vi "Tx Disable channel logic 1ch 4SPC.vi"(6 "ready for output":bool, 9 "input valid":bool, 10 "data in":u32[](array[numeric])=[0, 0, 0, 0, 0, 0, 0, 0, 0, 0, 0, 0, 0, 0, 0, 0]) -> (0 "enable new data":bool, 1 "output valid":bool, 2 "data out":u32[](array[numeric]))   [LabVIEW 2025, in "niUSRP Stream Control (DMA) v1 FPGA.lvclass"]
uses:
  niUSRP Stream Control (DMA) v1 FPGA.lvclass
  niUSRP Stream Control (DMA) v1 FPGA.lvclass/niUSRP Stream Control (DMA) v1 FPGA.ctl
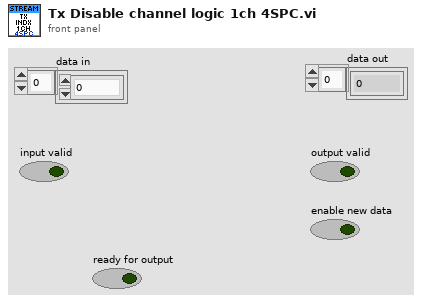
[diagram p1: front panel]
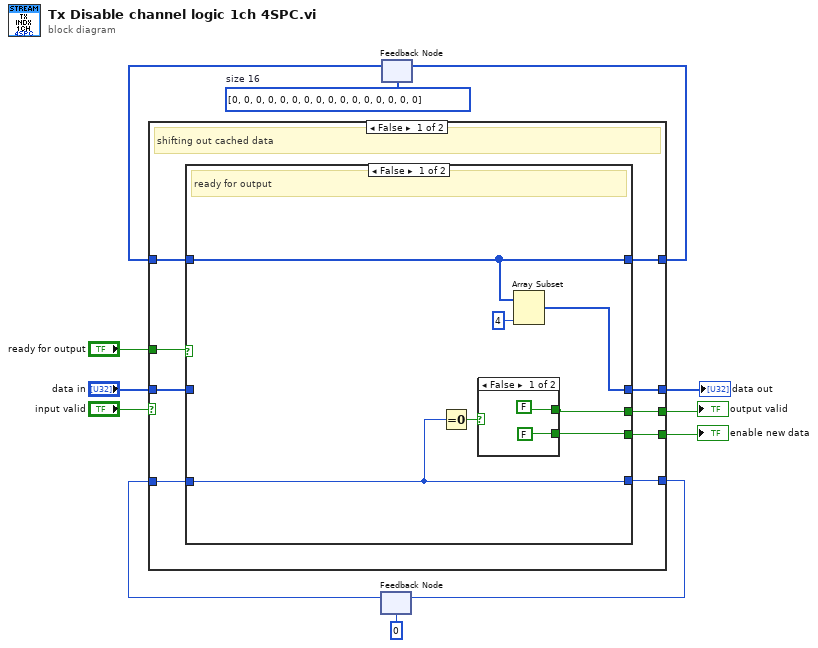
[diagram p0: block diagram]
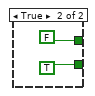
[diagram p2: hidden frame]
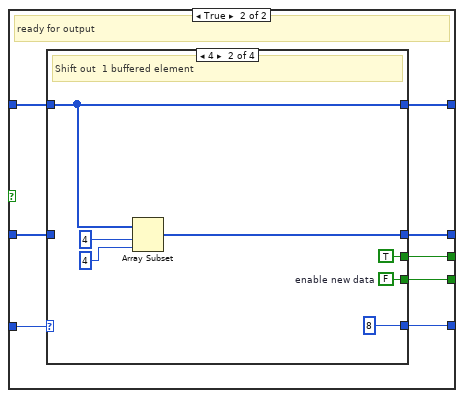
[diagram p3: hidden frame]
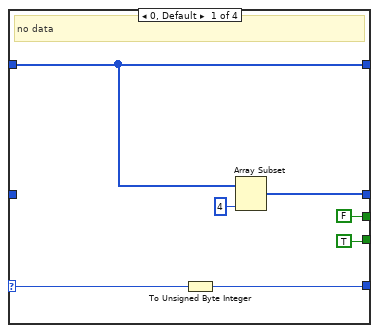
[diagram p4: hidden frame]
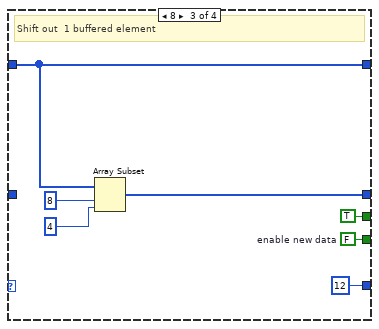
[diagram p5: hidden frame]
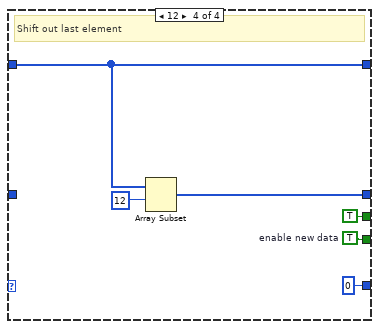
[diagram p6: hidden frame]
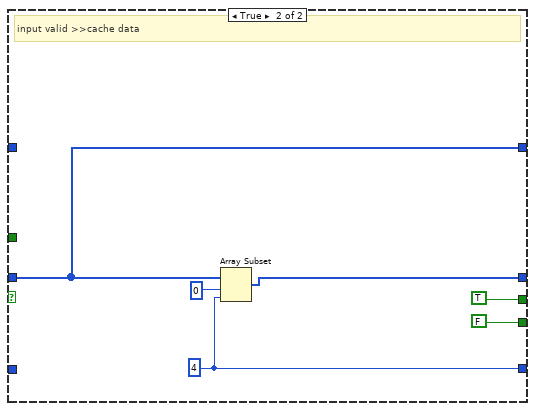
[diagram p7: hidden frame]
diagram:
  w6 = u32[] [0, 0, 0, 0, 0, 0, 0, 0, 0, 0, 0, 0, 0, 0, 0, 0]  # size 16
  n1 = feedback #1(u8 0) -> (w2:u8)
  n2 = feedback #2(w6) -> (w5:u32[])
  n3 = case shown="False" "input valid" {
    tunnel: [w21 TRUE] -> w12
    tunnel: [w20 FALSE ("enable new data")] -> w11
    tunnel: "data in" -> [w19 w70]
    tunnel: [w18 w71] -> w9
    tunnel: w5 -> [w17 _]
    tunnel: [w16 w70] -> w4
    tunnel: [w14 w69] -> w3
    tunnel: w2 -> [w15 _]
    tunnel: "ready for output" -> [w13 _]
    frame False {
      # "shifting out cached data"
      n4 = case shown="False" w13 {
        tunnel: [w26 w40] -> w21
        tunnel: [w25 w39] -> w20
        tunnel: w19 -> [_ w38]
        tunnel: [w22 w37] -> w18
        tunnel: w17 -> [w23 w36]
        tunnel: [w23 w35] -> w16
        tunnel: w15 -> [w27 w34]
        tunnel: [w27 w33] -> w14
        frame False {
          # "ready for output"
          n5 = Equal To 0?(x=w27) -> (x = 0?=w28:bool)
          n6 = case shown="False" w28 {
            tunnel: [FALSE TRUE] -> w25
            tunnel: [FALSE FALSE] -> w26
            frame False {
            }
            frame True {
            }
          }
          n7 = Array Subset(array=w23, length=4) -> (w22:u32[])  [unwired: 1 in]
        }
        frame True {
          # "ready for output"
          n8 = case shown="4" w34 {
            selector: w34 -> [w46 _ _ _]
            tunnel: w38 -> [_ _ _ _]
            tunnel: [w41 u8 8 ("length") u8 12 ("x+y") u8 0] -> w33
            tunnel: [w42 w51 w58 w63] -> w37
            tunnel: [FALSE TRUE TRUE TRUE] -> w40
            tunnel: w36 -> [w43 w53 w60 w64]
            tunnel: [w43 w53 w60 w64] -> w35
            tunnel: [TRUE w52 w59 w65] -> w39
            frame 0, Default {
              # "no data"
              n9 = To Unsigned Byte Integer(number=w46) -> (unsigned 8bit integer=w41:u8)
              n10 = Array Subset(array=w43, length=4) -> (w42:u32[])  [unwired: 1 in]
            }
            frame 4 {
              w52 = FALSE  # enable new data
              # "Shift out  1 buffered element"
              n11 = Array Subset(array=w53, index=4 ("length"), length=4) -> (w51:u32[])
            }
            frame 8 {
              w59 = FALSE  # enable new data
              # "Shift out  1 buffered element"
              n12 = Array Subset(array=w60, index=8 ("length"), length=4) -> (w58:u32[])
            }
            frame 12 {
              w65 = TRUE  # enable new data
              # "Shift out last element"
              n13 = Array Subset(array=w64, index=12) -> (w63:u32[])  [unwired: 1 in]
            }
          }
        }
      }
    }
    frame True {
      w69 = u8 4 ("y")
      # "input valid >>cache data"
      n14 = Array Subset(array=w70, index=0, length=w69) -> (w71:u32[])
    }
  }
  "output valid" <- w12
  "enable new data" <- w11
  "data out" <- w9
  n15 = feedback-in #1(w3) -> ()
  n16 = feedback-in #2(w4) -> ()
